vi "DSF.Shared.Configuration.Framework.Get Transfer Configurations.vi"(11 "Framework Configuration in":refnum<class "DSF.Shared.Configuration.Framework.lvclass">) -> (2 "Transfer Configurations":refnum<class "DSF.Shared.Configuration.Transfer.lvclass">[](array[class]), 3 "Framework Configuration out":refnum<class "DSF.Shared.Configuration.Framework.lvclass">)   [LabVIEW 2017, in "DSF.Shared.lvlib" / "DSF.Shared.Configuration.Framework.lvclass"]
uses:
  DSF.Shared.Configuration.Framework.lvclass
  Transfer/DSF.Shared.Configuration.Transfer.lvclass
  DSF.Shared.Configuration.Framework.lvclass/DSF.Shared.Configuration.Framework.ctl
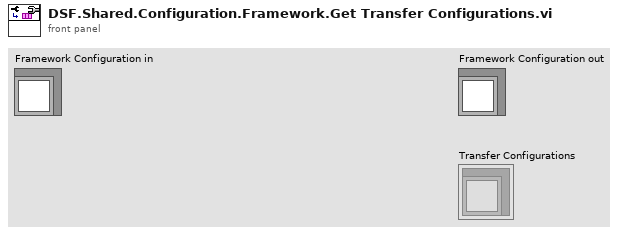
[diagram p1: front panel]
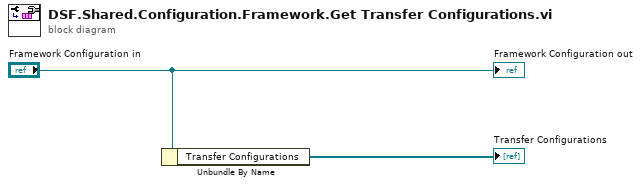
[diagram p0: block diagram]
diagram:
  n1 = Unbundle By Name("Framework Configuration in") -> ("Transfer Configurations"=→"Transfer Configurations":refnum<class "DSF.Shared.Configuration.Transfer.lvclass">[])
  "Framework Configuration out" <- "Framework Configuration in"
